vi "Initialize.vi"(8 "error IO":errorcluster, 10 "Software version":string="v1.14.0", 11 "Channel.lvclass":refnum<class "Channel.lvclass">) -> (0 "error IO 2":errorcluster, 1 "Initialization":bool, 3 "Channel.lvclass 2":refnum<class "Channel.lvclass">)   [LabVIEW 2018, in "Channel.lvclass"]
doc: "Initialize ACS"
uses:
  Channel.lvclass
  Channel.lvclass/Channel.ctl
  Header content/Header content.lvclass
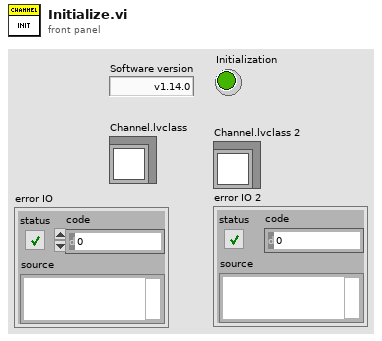
[diagram p1: front panel]
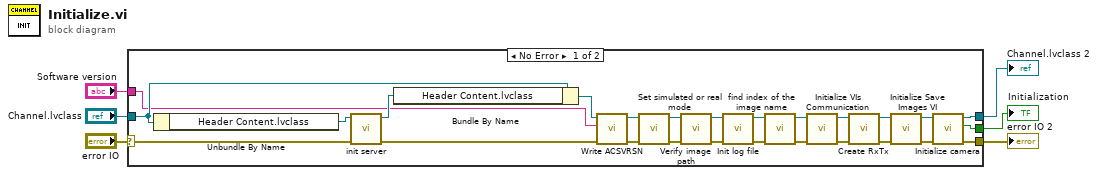
[diagram p0: block diagram]
diagram:
  n1 = case shown="No Error" "error IO" {
    selector: "error IO" -> [w19 w34]
    tunnel: [w7 w34] -> w3
    tunnel: [w8 w33] -> w4
    tunnel: "Channel.lvclass" -> [w18 w33]
    tunnel: [w22 _] -> w2
    tunnel: "Software version" -> [w9 _]
    frame No Error {
      n2 = Unbundle By Name(w18) -> ("Header Content.lvclass"=w21:refnum<class "Header content.lvclass">)
      n3 = call "init server.vi"("error in (no error)"=w19, "Header content in"=w21) -> ("error out"=w10:errorcluster, "Header content out"=w20:refnum<class "Header content.lvclass">)  [unwired: 8 in]
      n4 = Bundle By Name(cluster=w18, "Header Content.lvclass"=w20) -> (w13:refnum<class "Channel.lvclass">)
      n5 = call "Write ACSVRSN.vi"("error in (no error)"=w10, "ACSVRSN"=w9, "Channel in"=w13) -> ("error out"=w11:errorcluster, "Channel out"=w12:refnum<class "Channel.lvclass">)  [unwired: 7 in]
      n6 = call "Set simulated or real mode.vi"("error in (no error)"=w11, "Channel in"=w12) -> ("error out"=w16:errorcluster, "Channel out"=w17:refnum<class "Channel.lvclass">)  [unwired: 8 in]
      n7 = call "Verify image path.vi"("error in (no error)"=w16, "Channel in"=w17) -> ("error out"=w31:errorcluster, "Channel out"=w32:refnum<class "Channel.lvclass">)  [unwired: 8 in]
      n8 = call "Init log file.vi"("error in (no error)"=w31, "Channel in"=w32) -> ("error out"=w29:errorcluster, "Channel out"=w30:refnum<class "Channel.lvclass">)  [unwired: 8 in]
      n9 = call "find index of the image name.vi"("error in (no error)"=w29, "Channel in"=w30) -> ("error out"=w24:errorcluster, "Channel out"=w23:refnum<class "Channel.lvclass">)  [unwired: 8 in]
      n10 = call "Initialize VIs Communication.vi"("error in (no error)"=w24, "Channel in"=w23) -> ("error out"=w27:errorcluster, "Channel out"=w28:refnum<class "Channel.lvclass">)  [unwired: 8 in]
      n11 = call "Create RxTx.vi"("error in (no error)"=w27, "Channel in"=w28) -> ("error out"=w26:errorcluster, "Channel out"=w25:refnum<class "Channel.lvclass">)  [unwired: 8 in]
      n12 = call "Initialize Save Images VI.vi"("error in (no error)"=w26, "Channel in"=w25) -> ("error out"=w14:errorcluster, "Channel out"=w15:refnum<class "Channel.lvclass">)  [unwired: 8 in]
      n13 = call "Initialize camera.vi"("error in (no error)"=w14, "Channel in"=w15) -> ("error out"=w7:errorcluster, "Initialization"=w22:bool, "Channel out"=w8:refnum<class "Channel.lvclass">)  [unwired: 7 in]
    }
    frame Error {
    }
  }
  "Channel.lvclass 2" <- w4
  "error IO 2" <- w3
  "Initialization" <- w2
